vi "global1.vi"() -> ()   [LabVIEW 2015]
panel:
  out "card Number":dbl
  in  "Numeric":dbl
  in  "data":sgl[](array[numeric])
  in  "handler":u32
  in  "cardid":u32[](array[numeric])
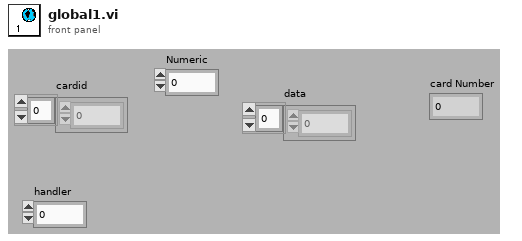
[diagram p1: front panel]
diagram:
